vi "Read configuration.vi"(8 "error in":errorcluster, 11 "bin datalogger editor node in":refnum<class "Binary datalogger editor node.lvclass">) -> (0 "error out":errorcluster, 2 "configuration":refnum<class "NISE_CEF_serializable configuration.lvclass">, 3 "bin datalogger editor node out":refnum<class "Binary datalogger editor node.lvclass">)   [LabVIEW 2013, in "Binary datalogger editor node.lvclass"]
uses:
  Binary datalogger editor node.lvclass
  <vilib>/NI/Configuration Framework/serializable configuration/NISE_CEF_serializable configuration.lvclass
  Binary datalogger editor node.lvclass/Binary datalogger editor node.ctl
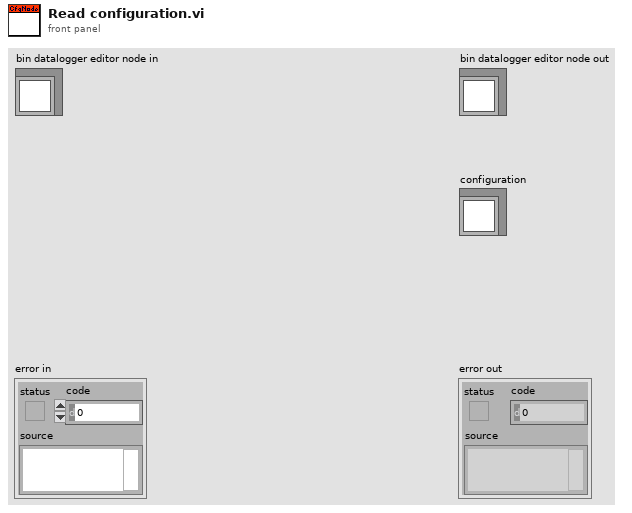
[diagram p1: front panel]
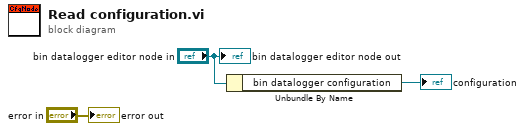
[diagram p0: block diagram]
diagram:
  n1 = Unbundle By Name("bin datalogger editor node in") -> ("bin datalogger configuration"=→"configuration":refnum<class "Binary datalogger configuration.lvclass">)
  "error out" <- "error in"
  "bin datalogger editor node out" <- "bin datalogger editor node in"
